vi "Subscribe.vi"(8 "error in (no error)":errorcluster, 10 "Subscription Request":refnum<class "SubscriptionRequest.lvclass">, 11 "Mediator In":refnum<class "Mediator.lvclass">) -> (0 "error out":errorcluster, 3 "Mediator Out":refnum<class "Mediator.lvclass">)   [LabVIEW 2015, in "Mediator.lvlib" / "Mediator.lvclass"]
doc: "<License>\nCopyright © 2017 Composed Systems, LLC | All rights reserved\nwww.composed.io\n\nAuthor: Ethan Stern <ethan.stern@composed.io>\n\nThis software is provided \"AS IS\" WITHOUT WARRANTIES, either express or implied, AND IS FOR EDUCATIONAL PURPOSES ONLY.\n</License>"
uses:
  Mediator.lvclass
  IMediator/SubscriptionRequest/SubscriptionRequest.lvclass
  Mediator.lvclass/Mediator.ctl
  IMediator/SubscriptionRequest/SubscriptionRequest.lvclass/SubscriptionRequest.ctl
  Topic Messages/Add Topic Subscriber Msg/Add Topic Subscriber Msg.lvclass/Add Topic Subscriber Msg.ctl
  <vilib>/ActorFramework/Message Enqueuer/Message Enqueuer.lvclass/Message Enqueuer.ctl
  <vilib>/ActorFramework/Message Enqueuer/Enqueue.vi
  <vilib>/ActorFramework/Message Priority Queue/Priority Enqueue.vi
  Topic Messages/Add Topic Subscriber Msg/Add Topic Subscriber Msg.lvclass
  TopicLookupTable/TopicLookupTable.lvclass
panel:
  # "What does subscriber want? (Datum Name and Type)\nHow does it get sent? (Transport)\nUnder what conditions? (SubscriptionPolicy)"
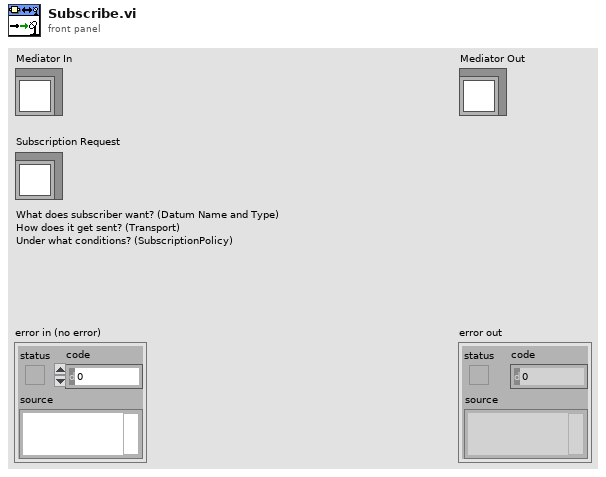
[diagram p1: front panel]
types:
  T1 = typedef "IMediator.lvlib/ISubscriptionPolicy.lvclass/ISubscriptionPolicy Reference.ctl" = refnum<data-value>
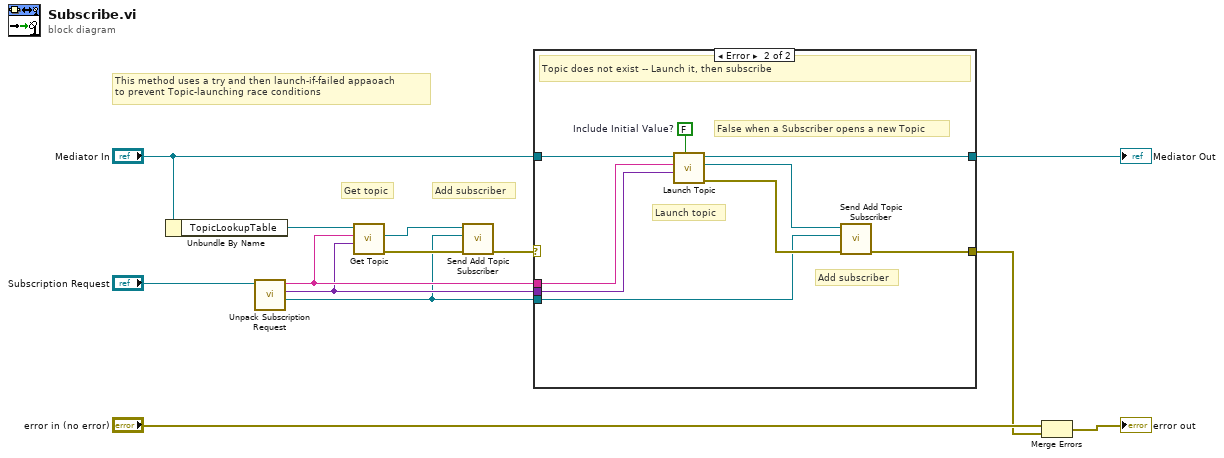
[diagram p0: block diagram]
diagram:
  # "This method uses a try and then launch-if-failed appaoach\nto prevent Topic-launching race conditions"
  # "Add subscriber"
  # "Get topic"
  n1 = Unbundle By Name("Mediator In") -> ("TopicLookupTable"=w2:refnum<data-value>)
  n2 = call "Unpack Subscription Request.vi"("SubscriptionRequest"="Subscription Request") -> ("Subscription Policy"=w1:T1, "Type"=w5:variant, "Datum Name"=w6:string)  [unwired: 8 in]
  n3 = call "Get Topic.vi"("Topic Type"=w5, "Topic Name"=w6, "TopicLookupTable"=w2) -> ("error out"=w7:errorcluster, "Topic Enqueuer"=w11:refnum<class "Message Enqueuer.lvclass">)  [unwired: 6 in, 1 out]
  n4 = call "Send Add Topic Subscriber.vi"("error in (no error)"=w7, "Subscription Policy"=w1, "Message Enqueuer"=w11) -> ("error out"=w9:errorcluster)  [unwired: 7 in, 1 out]
  n5 = case shown="Error" w9 {
    selector: w9 -> [w14 _]
    tunnel: "Mediator In" -> [w15 w19]
    tunnel: [w15 w23] -> w3
    tunnel: w6 -> [_ w18]
    tunnel: w5 -> [_ w17]
    tunnel: [w14 w24] -> w8
    tunnel: w1 -> [_ w20]
    frame No Error {
      # "Topic exists -- Subscribe OK"
    }
    frame Error {
      w16 = FALSE  # Include Initial Value?
      # "False when a Subscriber opens a new Topic"
      # "Launch topic"
      # "Add subscriber"
      # "Topic does not exist -- Launch it, then subscribe"
      n6 = call "Launch Topic.vi"("Include Initial Value? (F)"=w16, "Type"=w17, "Datum Name"=w18, "Mediator in"=w19) -> ("error out"=w21:errorcluster, "New Topic Enqueuer"=w22:refnum<class "Message Enqueuer.lvclass">, "Mediator out"=w23:refnum<class "Mediator.lvclass">)  [unwired: 5 in]
      n7 = call "Send Add Topic Subscriber.vi"("error in (no error)"=w21, "Subscription Policy"=w20, "Message Enqueuer"=w22) -> ("error out"=w24:errorcluster)  [unwired: 7 in, 1 out]
    }
  }
  "Mediator Out" <- w3
  n8 = Merge Errors("error in (no error)", w8) -> (→"error out":errorcluster)
